vi "MSDateienSchicken.vi"(0 "Dateipfad:fromcriocmd":path, 1 "Speicherlänge":string, 3 "wie wird gespeichert?":u16, 5 "Dateipfad:fromcriordy":path, 9 "Datum/Zeit":string, 11 "Dateien fürs MS schicken?":bool, 12 "Zyklnum1ges":i32, 14 "Info":string) -> ()   [LabVIEW 2010]
uses:
  <vilib>/addons/internet/NI_InternetTK_FTP_VIs.lvlib
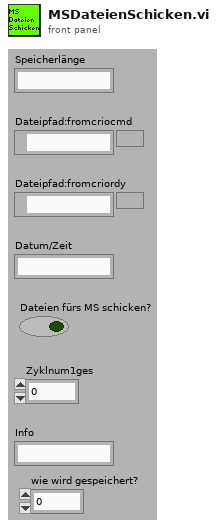
[diagram p1: front panel]
types:
  T1 = enum16{"open", "replace", "create", "open or create", "replace or create", "replace or create with confirmation"}
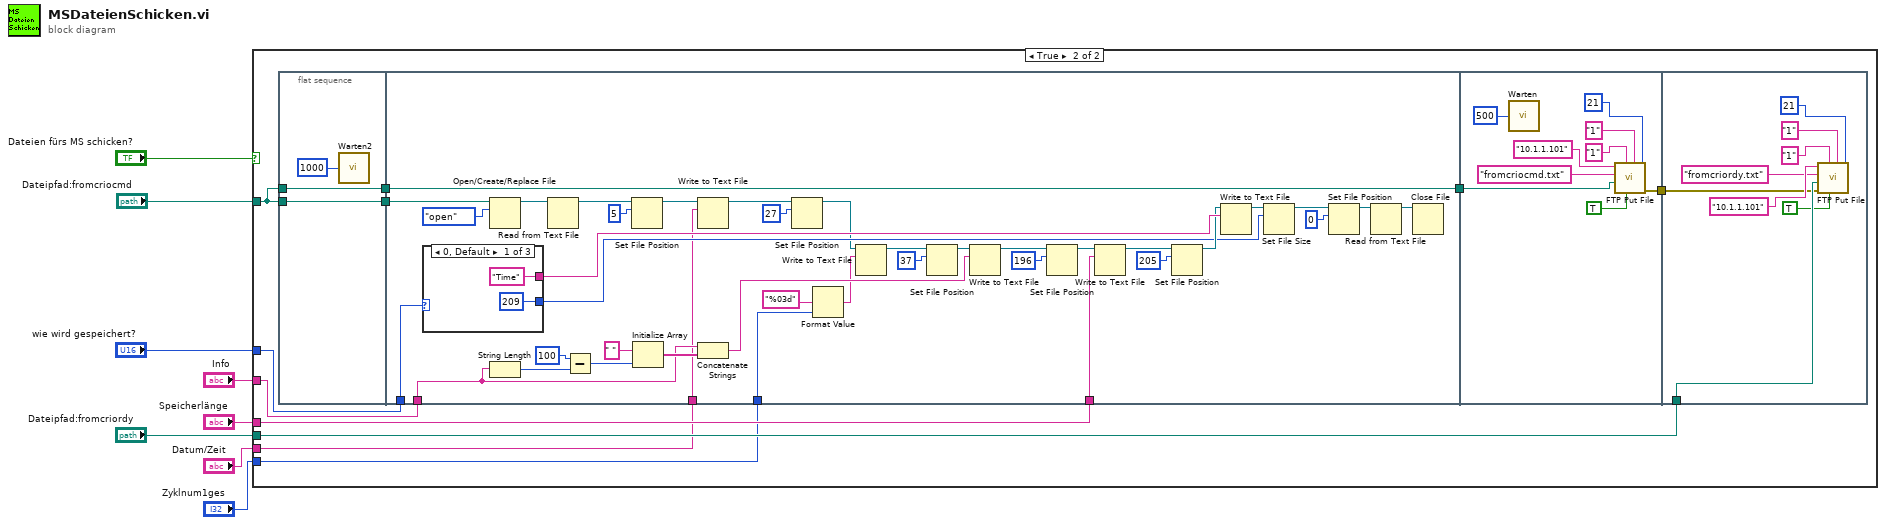
[diagram p0: block diagram]
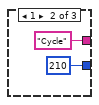
[diagram p3: hidden frame]
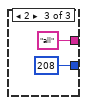
[diagram p4: hidden frame]
diagram:
  n1 = case shown="True" "Dateien fürs MS schicken?" {
    tunnel: "Dateipfad:fromcriordy" -> [_ w19]
    tunnel: "Dateipfad:fromcriocmd" -> [_ w9]
    tunnel: "wie wird gespeichert?" -> [_ w14]
    tunnel: "Speicherlänge" -> [_ w13]
    tunnel: "Info" -> [_ w12]
    tunnel: "Datum/Zeit" -> [_ w11]
    tunnel: "Zyklnum1ges" -> [_ w10]
    frame False {
    }
    frame True {
      n2 = flat-sequence {
        tunnel: w9 -> [w21]
        tunnel: w9 -> [w22]
        tunnel: [w22] -> w16
        tunnel: [w21] -> w15
        tunnel: [w61] -> w17
        tunnel: w16 -> [w61]
        tunnel: w15 -> [w28]
        tunnel: w14 -> [w27]
        tunnel: w13 -> [w26]
        tunnel: w12 -> [w25]
        tunnel: w11 -> [w24]
        tunnel: w10 -> [w23]
        tunnel: [w68] -> w18
        tunnel: w17 -> [w73]
        tunnel: w19 -> [w81]
        tunnel: w18 -> [w77]
        frame #0 {
          n3 = call "Warten2"("Count(mSec)"=u32 1000 ("Zu wartende ms")) -> ()  [unwired: 1 out]
        }
        frame #1 {
          n4 = case shown="0, Default" w27 {
            tunnel: ["Time" "Cycle" "all"] -> w52
            tunnel: [i64 209 ("Größe (in Byte)") i64 210 ("Größe (in Byte)") i64 208 ("Größe (in Byte)")] -> w45
            frame 0, Default {
            }
            frame 1 {
            }
            frame 2 {
            }
          }
          n5 = Open/Create/Replace File(file path (use dialog)=w28, operation (0:open)=T1."open" ("Operation (0:Öffnen)")) -> (refnum out=w31:refnum<file>)  [unwired: 4 in, 2 out]
          n6 = String Length(string=w25) -> (length=w55:i32)
          n7 = Read from Text File(file (use dialog)=w31) -> (refnum out=w32:refnum<file>)  [unwired: 3 in, 3 out]
          n8 = Subtract(x=100, y=w55) -> (x-y=w57:i32)
          n9 = Set File Position(offset (in bytes) (0)=i64 5 ("Offset (in Byte) (0)"), refnum=w32) -> (refnum out=w38:refnum<file>)  [unwired: 2 in, 1 out]
          n10 = Initialize Array(" ", w57) -> (w59:string[])
          n11 = Write to Text File(file (use dialog)=w38, text=w24) -> (refnum out=w40:refnum<file>)  [unwired: 2 in, 2 out]
          n12 = Concatenate Strings(w25, w59) -> (w60:string)
          n13 = Set File Position(offset (in bytes) (0)=i64 27 ("Offset (in Byte) (0)"), refnum=w40) -> (refnum out=w39:refnum<file>)  [unwired: 2 in, 1 out]
          n14 = Format Value(format string="%03d" ("Format-String"), value (0)=w23) -> (output string=w54:string)  [unwired: 1 in]
          n15 = Write to Text File(file (use dialog)=w39, text=w54) -> (refnum out=w41:refnum<file>)  [unwired: 2 in, 2 out]
          n16 = Set File Position(offset (in bytes) (0)=i64 37 ("Offset (in Byte) (0)"), refnum=w41) -> (refnum out=w42:refnum<file>)  [unwired: 2 in, 1 out]
          n17 = Write to Text File(file (use dialog)=w42, text=w60) -> (refnum out=w43:refnum<file>)  [unwired: 2 in, 2 out]
          n18 = Set File Position(offset (in bytes) (0)=i64 196 ("Offset (in Byte) (0)"), refnum=w43) -> (refnum out=w44:refnum<file>)  [unwired: 2 in, 1 out]
          n19 = Write to Text File(file (use dialog)=w44, text=w26) -> (refnum out=w50:refnum<file>)  [unwired: 2 in, 2 out]
          n20 = Set File Position(offset (in bytes) (0)=i64 205 ("Offset (in Byte) (0)"), refnum=w50) -> (refnum out=w49:refnum<file>)  [unwired: 2 in, 1 out]
          n21 = Write to Text File(file (use dialog)=w49, text=w52) -> (refnum out=w51:refnum<file>)  [unwired: 2 in, 2 out]
          n22 = Set File Size(6:w45, 7:w51) -> (3:w46:refnum<file>)  [unwired: 1 in, 1 out]
          n23 = Set File Position(offset (in bytes) (0)=i64 0 ("Offset (in Byte) (0)"), refnum=w46) -> (refnum out=w37:refnum<file>)  [unwired: 2 in, 1 out]
          n24 = Read from Text File(file (use dialog)=w37) -> (refnum out=w47:refnum<file>)  [unwired: 3 in, 3 out]
          n25 = Close File(refnum=w47) -> ()  [unwired: 1 in, 2 out]
        }
        frame #2 {
          n26 = call "Warten"("Count(mSec)"=u32 500 ("Zu wartende ms")) -> ()  [unwired: 1 out]
          n27 = call <vilib>:"FTP Put File.vi"("remote port (21)"=u16 21, "password"="1" ("user"), "binary (F)"=TRUE, "user"="1", "local path"=w73, "remote path"="fromcriocmd.txt", "host"="10.1.1.101") -> ("error out"=w68:errorcluster)  [unwired: 3 in, 1 out]
        }
        frame #3 {
          n28 = call <vilib>:"FTP Put File.vi"("remote port (21)"=u16 21, "password"="1" ("user"), "binary (F)"=TRUE, "user"="1", "error in (no error)"=w77, "local path"=w81, "remote path"="fromcriordy.txt", "host"="10.1.1.101") -> ()  [unwired: 2 in, 2 out]
        }
      }
    }
  }
